vi "ReadCase.vi"(8 "error in (no error)":errorcluster, 11 "Current path":path) -> (0 "error out":errorcluster, 3 "Case number":string)   [LabVIEW 2020]
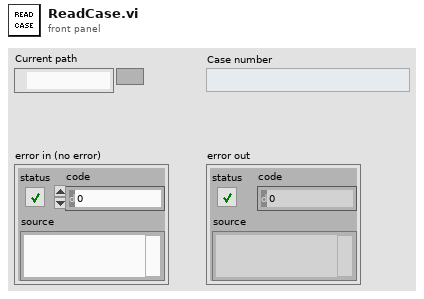
[diagram p1: front panel]
types:
  T1 = enum16{"open", "replace", "create", "open or create", "replace or create", "replace or create with confirmation"}
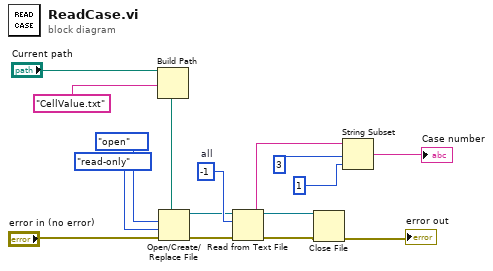
[diagram p0: block diagram]
diagram:
  w12 = -1  # all
  n1 = Build Path(base path="Current path", name or relative path="CellValue.txt") -> (appended path=w9:path)
  n2 = Open/Create/Replace File(file path (use dialog)=w9, error in="error in (no error)", operation (0:open)=T1."open", access (0:read/write)=enum16{"read/write", "read-only", "write-only"}."read-only") -> (refnum out=w10:refnum<file>, error out=w11:errorcluster)  [unwired: 2 in, 1 out]
  n3 = Read from Text File(file (use dialog)=w10, count=w12, error in=w11) -> (refnum out=w13:refnum<file>, text=w4:string, error out=w14:errorcluster)  [unwired: 1 in, 1 out]
  n4 = Close File(refnum=w13, error in=w14) -> (error out=→"error out":errorcluster)  [unwired: 1 out]
  n5 = String Subset(string=w4, offset (0)=3, length (rest)=1) -> (substring=→"Case number":string)
